vi "判定转范围.vi"(11 "判定":string[][](array[string])) -> (3 "范围":string)   [LabVIEW 2018]
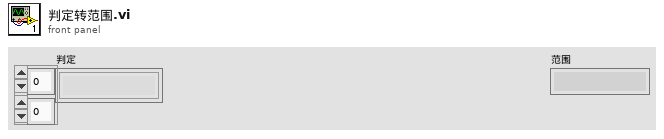
[diagram p1: front panel]
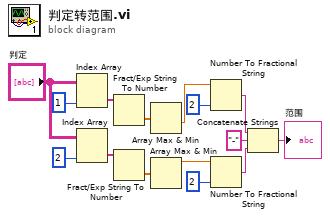
[diagram p0: block diagram]
diagram:
  n1 = Index Array(array="判定", index (col)=1 ("索引 (行)")) -> (element=w13:string[])  [unwired: 1 in]
  n2 = Index Array(array="判定", index (col)=2 ("禁用的索引 (列)")) -> (element=w11:string[])  [unwired: 1 in]
  n3 = Fract/Exp String To Number(string=w13) -> (number=w12:dbl[])  [unwired: 3 in, 1 out]
  n4 = Fract/Exp String To Number(string=w11) -> (number=w10:dbl[])  [unwired: 3 in, 1 out]
  n5 = Array Max & Min(array=w12) -> (min value=w9:dbl)  [unwired: 3 out]
  n6 = Array Max & Min(array=w10) -> (max value=w8:dbl)  [unwired: 3 out]
  n7 = Number To Fractional String(number=w9, precision (6)=i16 2 ("精度(6)")) -> (F-format string=w7:string)  [unwired: 2 in]
  n8 = Number To Fractional String(number=w8, precision (6)=i16 2 ("精度(6)")) -> (F-format string=w5:string)  [unwired: 2 in]
  n9 = Concatenate Strings(w7, "-" ("字符串"), w5) -> (→"范围":string)
